vi "M2.vi"(1 "x":i32) -> (0 "64bit integer":i64)   [LabVIEW 2012]
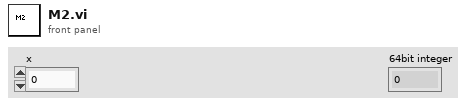
[diagram p1: front panel]
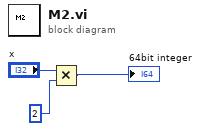
[diagram p0: block diagram]
diagram:
  n1 = Multiply(x="x", y=2) -> (x*y=→"64bit integer":i32)
